vi "Transformation Matrix to Pose.vi"(8 "error in (no error)":errorcluster, 11 "4x4 Transformation Matrix":T1) -> (0 "error out":errorcluster, 3 "Pose":T2)   [LabVIEW 2020, in "ar.lvlib"]
doc: "Convert a 4x4 Transformation Matrix to a 3D Pose."
uses:
  ar.lvlib
  Pose.ctl
  rvec.ctl
  tvec.ctl
  <vilib>/Analysis/Matrix/Datatypes/RealMatrix.ctl
  Rodrigues (RMat To RVec).vi
  <vilib>/Utility/error.llb/Error Cluster From Error Code.vi
  <vilib>/Analysis/Matrix/NI_Matrix.lvlib
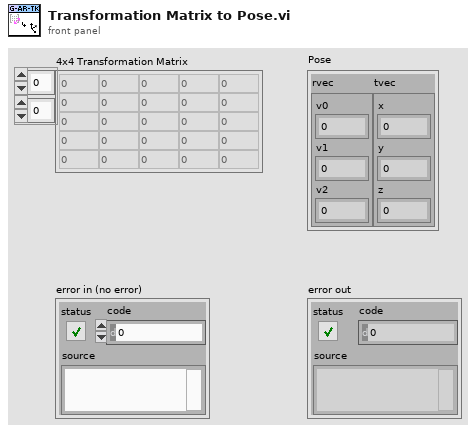
[diagram p1: front panel]
types:
  T1 = typedef "NI_Matrix.lvlib/RealMatrix.ctl" = dbl[][]
  T2 = typedef "ar.lvlib/Pose.ctl" = cluster{"rvec":T3, "tvec":T4}
  T3 = typedef "ar.lvlib/rvec.ctl" = cluster{"v0":dbl, "v1":dbl, "v2":dbl}
  T4 = typedef "ar.lvlib/tvec.ctl" = cluster{"x":dbl, "y":dbl, "z":dbl}
  T5 = cluster{"4x4 Transformation Matrix[0]":dbl, "4x4 Transformation Matrix[1]":dbl, "4x4 Transformation Matrix[2]":dbl}
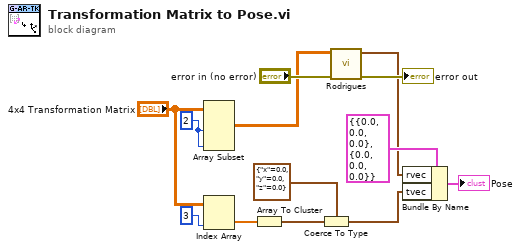
[diagram p0: block diagram]
diagram:
  w11 = 2 ("row N")
  n1 = Array Subset(array="4x4 Transformation Matrix", length (row)=w11, length (col)=w11) -> (w10:T1)  [unwired: 2 in]
  n2 = Index Array(array="4x4 Transformation Matrix", index (col)=3 ("disabled index (col)")) -> (element=w7:dbl[])  [unwired: 1 in]
  n3 = Array To Cluster(array=w7) -> (cluster=w3:T5)
  n4 = Coerce To Type(0:w3, 1:T4 {"x"=0.0, "y"=0.0, "z"=0.0} ("tvec")) -> (2:w2:T4)
  n5 = call-poly "Rodrigues.vi"("error in (no error)"="error in (no error)", "Rotation Matrix"=w10) -> ("error out"=→"error out":errorcluster, "rvec"=w4:T3)  [unwired: 8 in]
  n6 = Bundle By Name(cluster=T2 {"rvec"={"v0"=0.0, "v1"=0.0, "v2"=0.0}, "tvec"={"x"=0.0, "y"=0.0, "z"=0.0}} ("Pose"), "rvec"=w4, "tvec"=w2) -> (→"Pose":T2)
